vi "RecordingDisplay_171213.vi"(0 "TrackLength":dbl, 1 "Segments":bool, 2 "NormalMousebackgraound":picture, 4 "BackgroundSegments":picture, 6 "X":i32, 7 "Y":i32, 8 "i":i32, 9 "X in":i32[](array[numeric]), 10 "Angle":dbl, 11 "Y in":i32[](array[numeric])) -> (12 "X out":i32[](array[numeric]), 13 "Y out":i32[](array[numeric]), 19 "RecordingDisplay":picture)   [LabVIEW 2016]
uses:
  Globaltracker.vi
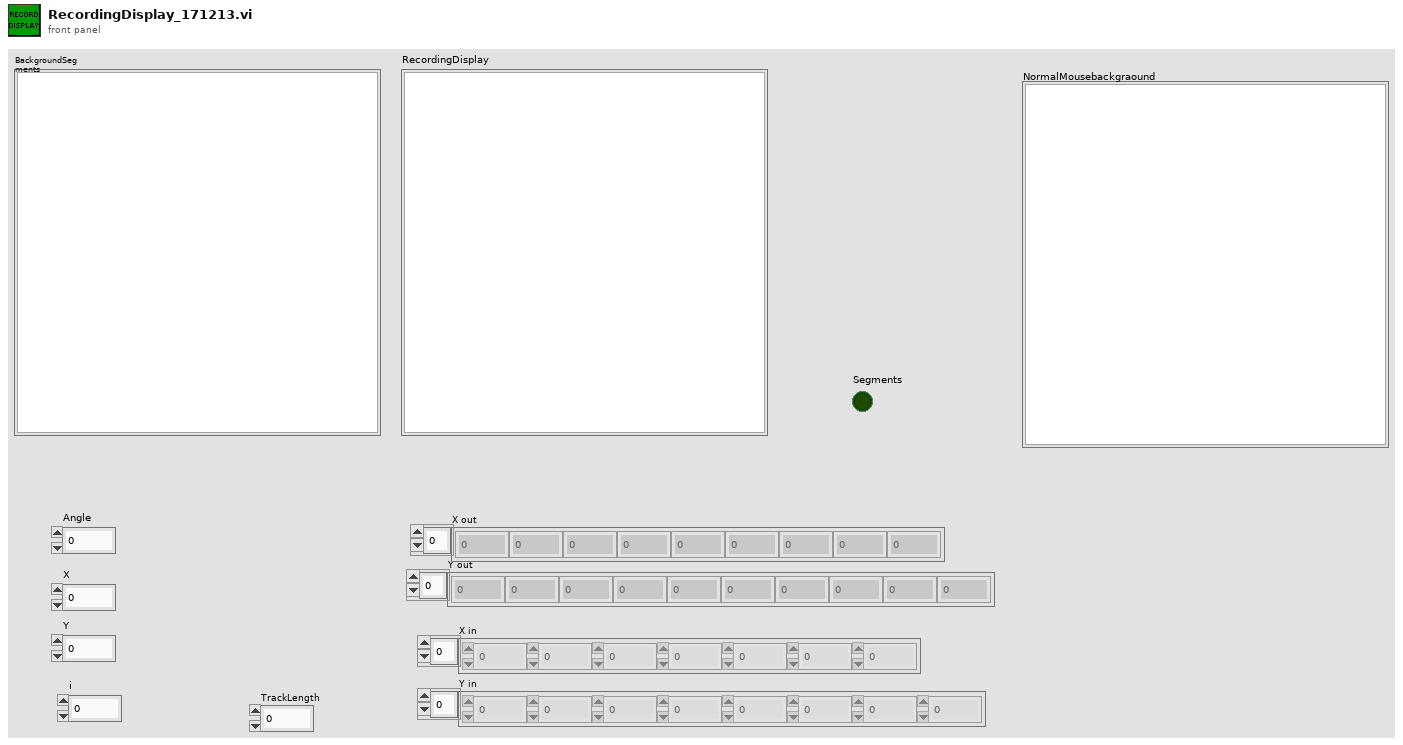
[diagram p1: front panel]
types:
  T1 = typedef "imagedata.ctl" = cluster{"image type":i32, "image depth":i32, "image":u8[], "mask":u8[], "colors":u32[], "Rectangle":cluster{"left":i16, "top":i16, "right":i16, "bottom":i16}}
  T2 = cluster{"left":i16, "top":i16, "right":i16, "bottom":i16}
  T3 = cluster{"image type":i32, "image depth":i32, "image":u8[], "mask":u8[], "colors":u32[], cluster{i32, i32, i32, i32}}
  T4 = cluster{"Width":u16, "Style":enum32{"Solid", "Dash", "Dot", "DashDot", "DashDotDot"}}
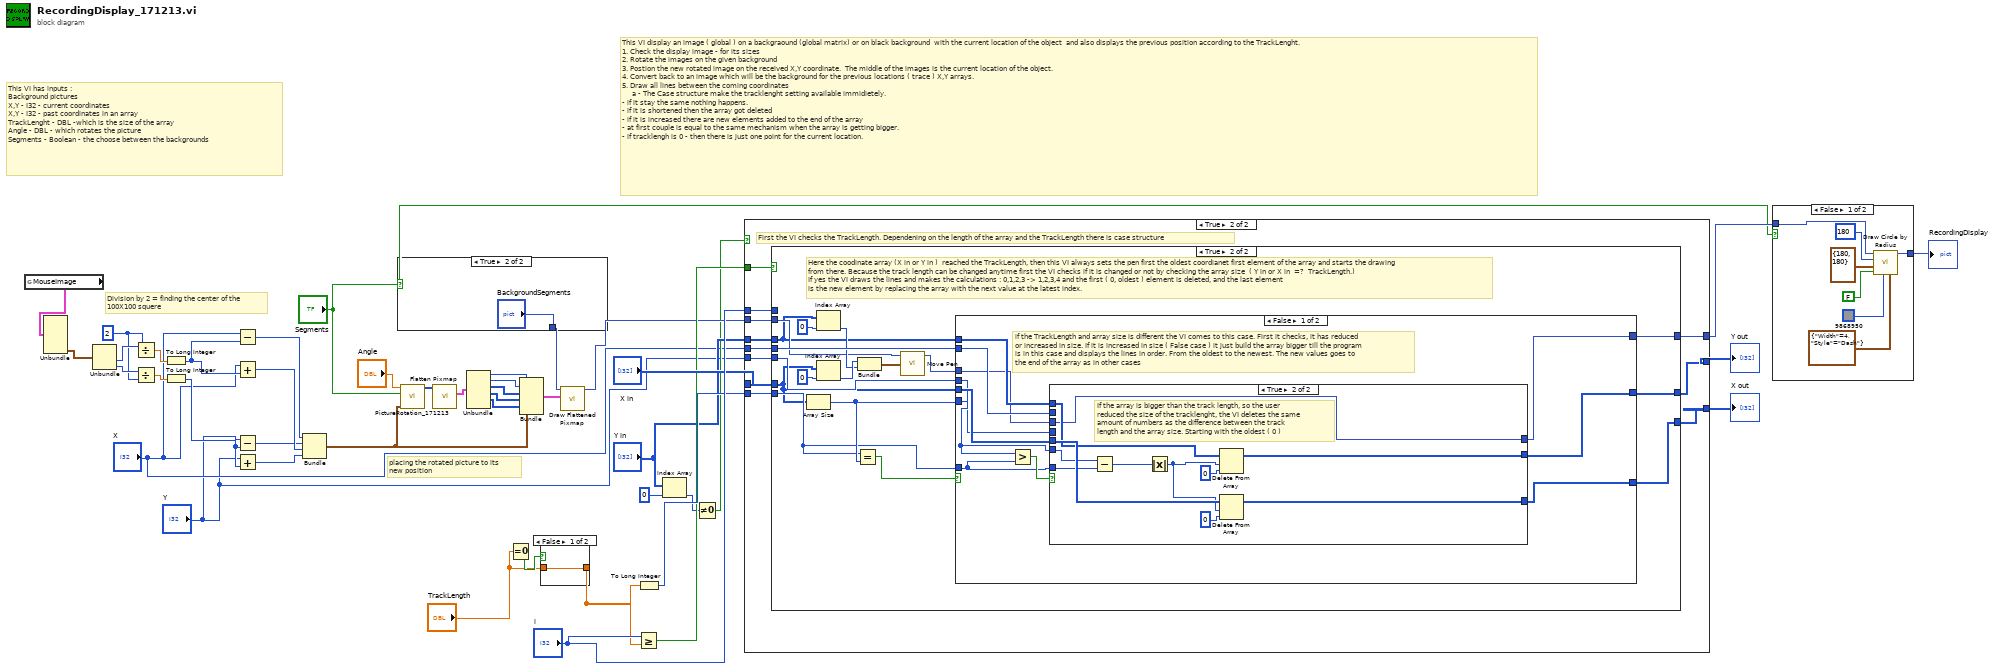
[diagram p0: block diagram]
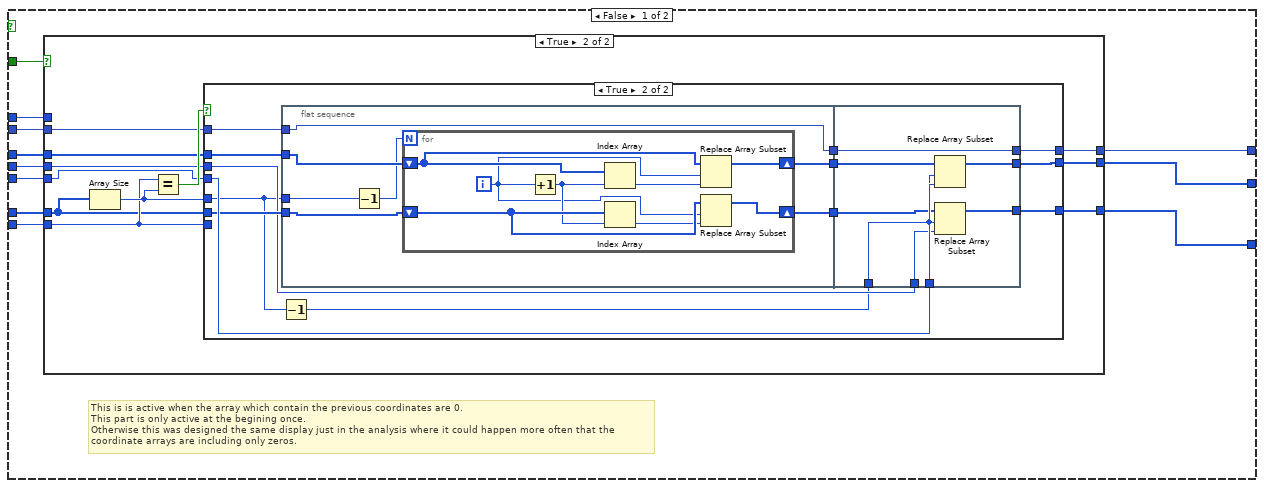
[diagram p2: hidden frame]
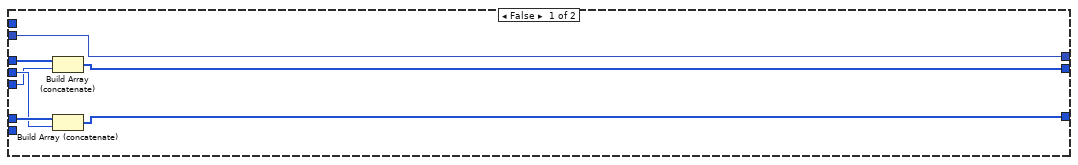
[diagram p3: hidden frame]
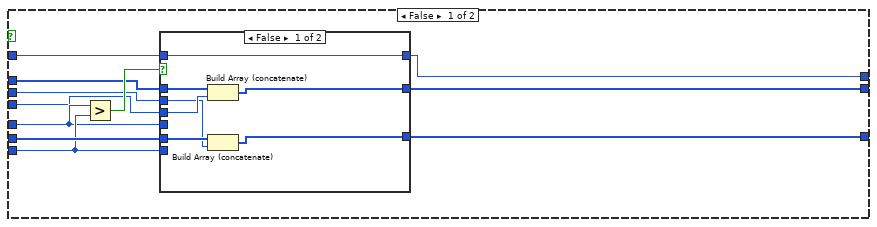
[diagram p4: hidden frame]
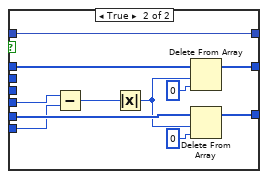
[diagram p5: hidden frame]
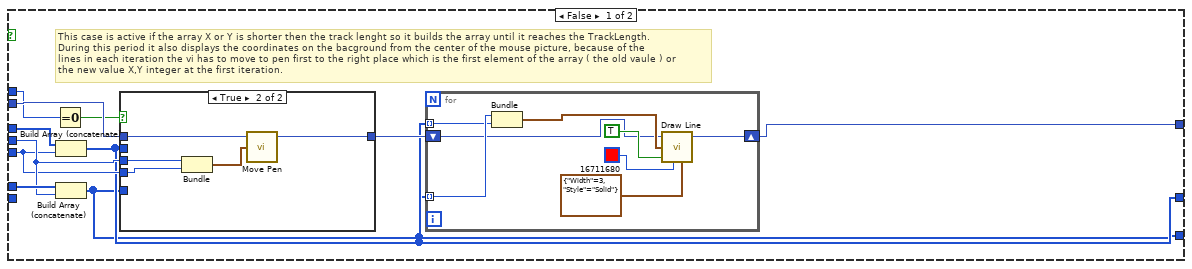
[diagram p6: hidden frame]
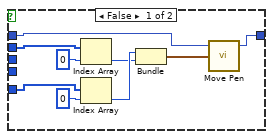
[diagram p7: hidden frame]
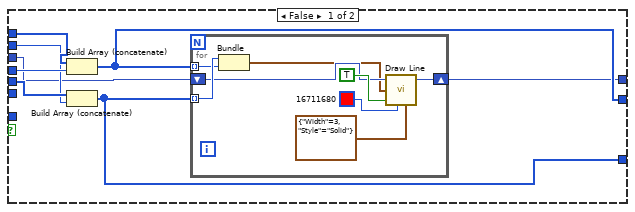
[diagram p8: hidden frame]
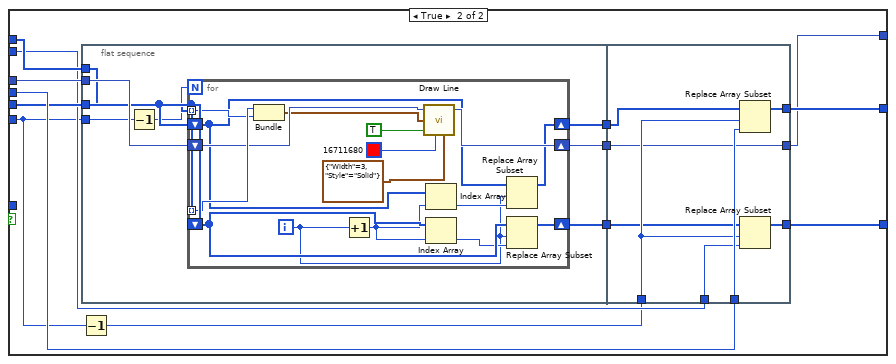
[diagram p9: hidden frame]
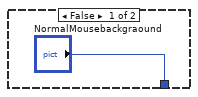
[diagram p10: hidden frame]
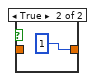
[diagram p11: hidden frame]
diagram:
  w17 = i16 2 ("y")
  # "placing the rotated picture to its \nnew position"
  # "Division by 2 = finding the center of the\n100X100 squere"
  # "This VI display an image ( global ) on a backgraound (global matrix) or on black background  with the current location of the object  and also displays the previous position according to the TrackLenght.\n1. Check the display image - for its sizes\n2. Rotate the images on the given background\n3. Postion the new rotated image on the received X,Y coordinate.  The middle of the images is the current location of the object.\n4. Convert back to an image which will be the background for the previous locations ( trace ) X,Y arrays. \n5. Draw all lines between the coming coordinates \n     a - The Case structure make the tracklenght setting available immidietely. \n- if it stay the same nothing happens.\n- if it is shortened then the array got deleted\n- if it is increased there are new elements added to the end of the array\n- at first couple is equal to the same mechanism when the array is getting bigger.\n- if tracklengh is 0 - then there is just one point for the current location."
  # "This VI has inputs : \nBackground pictures\nX,Y - I32 - current coordinates \nX,Y - I32 - past coordinates in an array \nTrackLenght - DBL -which is the size of the array\nAngle - DBL - which rotates the picture\nSegments - Boolean - the choose between the backgrounds"
  n1 = global read "Globaltracker.vi" "MouseImage"() -> (w21:T1)
  n2 = Unbundle(w21) -> ("Rectangle"=w20:T2)  [unwired: 5 out]
  n3 = Unbundle(w20) -> ("right"=w19:i16, "bottom"=w18:i16)  [unwired: 2 out]
  n4 = Divide(x=w19, y=w17) -> (x/y=w16:dbl)
  n5 = Divide(x=w18, y=w17) -> (x/y=w15:dbl)
  n6 = To Long Integer(number=w16) -> (32bit integer=w14:i32)
  n7 = To Long Integer(number=w15) -> (32bit integer=w13:i32)
  n8 = Subtract(x="X", y=w14) -> (x-y=w35:i32)
  n9 = Add(x="X", y=w14) -> (x+y=w34:i32)
  n10 = Subtract(x="Y", y=w13) -> (x-y=w32:i32)
  n11 = Add(x="Y", y=w13) -> (x+y=w33:i32)
  n12 = Bundle(w35, w32, w34, w33) -> (w24:cluster{i32, i32, i32, i32})  [unwired: 1 in]
  n13 = case shown="True" "Segments" {
    tunnel: ["NormalMousebackgraound" "BackgroundSegments"] -> w8
    frame False {
    }
    frame True {
    }
  }
  n14 = call "PictureRotation_171213.vi"("Cluster"=w24, "Segments"="Segments", "Angle"="Angle") -> ("Array"=w12:u32[][])  [unwired: 8 in]
  n15 = call <vilib>:"Flatten Pixmap.vi"("24-bit pixmap"=w12) -> ("image data"=w30:T1)  [unwired: 10 in]
  n16 = Unbundle(w30) -> ("image type"=w29:i32, "image depth"=w28:i32, "image"=w27:u8[], "mask"=w26:u8[], "colors"=w25:u32[])  [unwired: 1 out]
  n17 = Equal To 0?(x="TrackLength") -> (x = 0?=w42:bool)
  n18 = Bundle("image type"=w29, "image depth"=w28, "image"=w27, "mask"=w26, "colors"=w25, w24) -> (w23:T3)  [unwired: 1 in]
  n19 = case shown="False" w42 {
    tunnel: "TrackLength" -> [w46 _]
    tunnel: [w46 1] -> w7
    frame False {
    }
    frame True {
    }
  }
  n20 = call <vilib>:"Draw Flattened Pixmap.vi"("image data"=w23, "picture"=w8) -> ("new picture"=w22:picture)  [unwired: 7 in]
  n21 = Greater Or Equal?(x="i", y=w7) -> (x >= y?=w36:bool)
  n22 = To Long Integer(number=w7) -> (32bit integer=w40:i32)
  n23 = Index Array(array="Y in", index=0) -> (element=w5:i32)
  n24 = Not Equal To 0?(x=w5) -> (x != 0?=w3:bool)
  n25 = case shown="True" w3 {
    tunnel: "i" -> [w52 w152]
    tunnel: w40 -> [w53 w151]
    tunnel: "X in" -> [w57 w150]
    tunnel: [w48 w149] -> w38
    tunnel: [w49 w148] -> w37
    tunnel: w36 -> [w51 w147]
    tunnel: w22 -> [w58 w146]
    tunnel: [w50 w145] -> w11
    tunnel: "X" -> [w55 w144]
    tunnel: "Y" -> [w54 w143]
    tunnel: "Y in" -> [w56 w142]
    frame False {
      # "This is is active when the array which contain the previous coordinates are 0. \nThis part is only active at the begining once.\nOtherwise this was designed the same display just in the analysis where it could happen more often that the \ncoordinate arrays are including only zeros."
      n26 = case shown="True" w51 {
        tunnel: [w59 w75] -> w50
        tunnel: w52 -> [_ _]
        tunnel: w53 -> [_ w72]
        tunnel: w54 -> [w62 w71]
        tunnel: [w60 w69] -> w49
        tunnel: [w61 w76] -> w48
        tunnel: w56 -> [w65 w68]
        tunnel: w57 -> [w64 w67]
        tunnel: w55 -> [w63 w70]
        tunnel: w58 -> [w59 w66]
        frame False {
          n27 = Build Array (concatenate)(w65, w62) -> (w61:i32[])
          n28 = Build Array (concatenate)(w64, w63) -> (w60:i32[])
        }
        frame True {
          n29 = Array Size(array=w67) -> (size(s)=w73:i32)
          n30 = Equal?(x=w72, y=w73) -> (x = y?=w74:bool)
          n31 = case shown="True" w74 {
            tunnel: [w86 w118] -> w69
            tunnel: [w85 w117] -> w76
            tunnel: w71 -> [w77 w116]
            tunnel: w67 -> [w84 w115]
            tunnel: w68 -> [w83 w114]
            tunnel: w66 -> [w79 w113]
            tunnel: [w78 w109] -> w75
            tunnel: w73 -> [w81 w108]
            tunnel: w72 -> [w82 _]
            tunnel: w70 -> [w80 w112]
            frame False {
              n32 = Greater?(x=w81, y=w82) -> (0:w87:bool)
              n33 = case shown="False" w87 {
                tunnel: [w89 w105] -> w86
                tunnel: [w90 w104] -> w85
                tunnel: w84 -> [w94 w103]
                tunnel: w83 -> [w93 w102]
                tunnel: w81 -> [_ w101]
                tunnel: w82 -> [_ w97]
                tunnel: w77 -> [w92 _]
                tunnel: w80 -> [w91 _]
                tunnel: w79 -> [w88 w98]
                tunnel: [w88 w98] -> w78
                frame False {
                  n34 = Build Array (concatenate)(w93, w92) -> (w90:i32[])
                  n35 = Build Array (concatenate)(w94, w91) -> (w89:i32[])
                }
                frame True {
                  n36 = Subtract(x=w101, y=w97) -> (x-y=w100:i32)
                  n37 = Absolute Value(x=w100) -> (abs(x)=w99:i32)
                  n38 = Delete From Array(array=w102, length=w99, index=0) -> (array with subset deleted=w104:i32[])  [unwired: 1 out]
                  n39 = Delete From Array(array=w103, length=w99, index=0) -> (array with subset deleted=w105:i32[])  [unwired: 1 out]
                }
              }
            }
            frame True {
              n40 = Decrement(x=w108) -> (x-1=w111:i32)
              n41 = flat-sequence {
                tunnel: w115 -> [w125]
                tunnel: w114 -> [w124]
                tunnel: w113 -> [w119]
                tunnel: [w119] -> w110
                tunnel: w108 -> [w123]
                tunnel: [w121] -> w107
                tunnel: [w120] -> w106
                tunnel: [w141] -> w118
                tunnel: [w140] -> w117
                tunnel: w116 -> [w139]
                tunnel: w112 -> [w138]
                tunnel: w111 -> [w137]
                tunnel: w110 -> [w136]
                tunnel: [w136] -> w109
                tunnel: w107 -> [w135]
                tunnel: w106 -> [w134]
                frame #0 {
                  n42 = Decrement(x=w123) -> (x-1=w122:i32)
                  n43 = for {
                    N: w122 -> [_]
                    shift-right: [w127] -> w121
                    shift-left: w125 -> [w133]
                    shift-right: [w126] -> w120
                    shift-left: w124 -> [w132]
                    i -> [w128]
                    n44 = Increment(x=w128) -> (x+1=w131:i32)
                    n45 = Index Array(array=w132, index=w131) -> (element=w129:i32)
                    n46 = Index Array(array=w133, index=w131) -> (element=w130:i32)
                    n47 = Replace Array Subset(array=w132, new element=w129, index=w128) -> (w126:i32[])
                    n48 = Replace Array Subset(array=w133, new element=w130, index=w128) -> (w127:i32[])
                  }
                }
                frame #1 {
                  n49 = Replace Array Subset(array=w134, new element=w139, index=w137) -> (w140:i32[])
                  n50 = Replace Array Subset(array=w135, new element=w138, index=w137) -> (w141:i32[])
                }
              }
            }
          }
        }
      }
    }
    frame True {
      # "First the VI checks the TrackLength. Dependening on the length of the array and the TrackLength there is case structure"
      n51 = case shown="True" w147 {
        tunnel: [w161 w201] -> w145
        tunnel: w152 -> [w156 _]
        tunnel: w151 -> [_ w198]
        tunnel: w143 -> [w158 w197]
        tunnel: [w153 w195] -> w148
        tunnel: [w154 w202] -> w149
        tunnel: w142 -> [w163 w187]
        tunnel: w150 -> [w162 w186]
        tunnel: w144 -> [w160 w196]
        tunnel: w146 -> [w159 w189]
        frame False {
          # "This case is active if the array X or Y is shorter then the track lenght so it builds the array until it reaches the TrackLength.\nDuring this period it also displays the coordinates on the bacground from the center of the mouse picture, because of the \nlines in each iteration the vi has to move to pen first to the right place which is the first element of the array ( the old vaule ) or \nthe new value X,Y integer at the first iteration."
          n52 = Equal To 0?(x=w156) -> (x = 0?=w157:bool)
          n53 = Build Array (concatenate)(w163, w158) -> (w154:i32[])
          n54 = Build Array (concatenate)(w162, w160) -> (w153:i32[])
          n55 = case shown="True" w157 {
            tunnel: w160 -> [_ w177]
            tunnel: w159 -> [w170 w176]
            tunnel: w158 -> [_ w175]
            tunnel: [w171 w173] -> w155
            tunnel: w154 -> [w169 _]
            tunnel: w153 -> [w168 _]
            frame False {
              n56 = Index Array(array=w169, index=0) -> (element=w164:i32)
              n57 = Index Array(array=w168, index=0) -> (element=w165:i32)
              n58 = Bundle("X"=w165, "Y"=w164) -> (w172:cluster{"X":i32, "Y":i32})  [unwired: 1 in]
              n59 = call <vilib>:"Move Pen.vi"("new position"=w172, "picture"=w170) -> ("new picture"=w171:picture)  [unwired: 3 in]
            }
            frame True {
              n60 = Bundle("X"=w177, "Y"=w175) -> (w174:cluster{"X":i32, "Y":i32})  [unwired: 1 in]
              n61 = call <vilib>:"Move Pen.vi"("new position"=w174, "picture"=w176) -> ("new picture"=w173:picture)  [unwired: 3 in]
            }
          }
          n62 = for {
            tunnel: w153 -> [w185] mode=indexing
            tunnel: w154 -> [w184] mode=indexing
            shift-right: [w179] -> w161
            shift-left: w155 -> [w178]
            n63 = Bundle("X"=w185, "Y"=w184) -> (w180:cluster{"X":i32, "Y":i32})  [unwired: 1 in]
            n64 = call <vilib>:"Draw Line.vi"("picture"=w178, "end point"=w180, "absolute coordinates?(T)"=TRUE, "color(black)"=u32 16711680, "pen"=T4 {"Width"=3, "Style"=enum."Solid"}) -> ("new picture"=w179:picture)  [unwired: 4 in]
          }
        }
        frame True {
          # "Here the coodinate array (X in or Y in )  reached the TrackLength, then this VI always sets the pen first the oldest coordianet first element of the array and starts the drawing \nfrom there. Because the track length can be changed anytime first the VI checks if it is changed or not by checking the array size  ( Y in or X in  =?  TrackLength.)\nIf yes the VI draws the lines and makes the calculations : 0,1,2,3 -> 1,2,3,4 and the first ( 0, oldest ) element is deleted, and the last element\nis the new element by replacing the array with the next value at the latest index."
          n65 = Array Size(array=w186) -> (size(s)=w199:i32)
          n66 = Index Array(array=w187, index=0) -> (element=w192:i32)
          n67 = Index Array(array=w186, index=0) -> (element=w193:i32)
          n68 = Equal?(x=w198, y=w199) -> (x = y?=w200:bool)
          n69 = Bundle(w193, w192) -> (w194:cluster{i32, i32})  [unwired: 1 in]
          n70 = call <vilib>:"Move Pen.vi"("new position"=w194, "picture"=w189) -> ("new picture"=w188:picture)  [unwired: 3 in]
          n71 = case shown="False" w200 {
            tunnel: [w212 w253] -> w195
            tunnel: [w211 w252] -> w202
            tunnel: w197 -> [w203 w251]
            tunnel: w186 -> [w210 w250]
            tunnel: w187 -> [w209 w249]
            tunnel: w188 -> [w205 w248]
            tunnel: [w204 w244] -> w201
            tunnel: w199 -> [w207 w243]
            tunnel: w198 -> [w208 _]
            tunnel: w196 -> [w206 w247]
            frame False {
              # "if the TrackLength and array size is different the VI comes to this case. First it checks, it has reduced\nor increased in size. If it is increased in size ( False case ) it just build the array bigger till the program\nis in this case and displays the lines in order. From the oldest to the newest. The new values goes to\nthe end of the array as in other cases"
              n72 = Greater?(x=w207, y=w208) -> (0:w213:bool)
              n73 = case shown="True" w213 {
                tunnel: [w216 w240] -> w212
                tunnel: [w217 w239] -> w211
                tunnel: w210 -> [w221 w238]
                tunnel: w209 -> [w220 w237]
                tunnel: w207 -> [_ w236]
                tunnel: w208 -> [_ w232]
                tunnel: w203 -> [w219 _]
                tunnel: w206 -> [w218 _]
                tunnel: w205 -> [w215 w233]
                tunnel: [w214 w233] -> w204
                frame False {
                  n74 = Build Array (concatenate)(w220, w219) -> (w217:i32[])
                  n75 = Build Array (concatenate)(w221, w218) -> (w216:i32[])
                  n76 = for {
                    tunnel: w216 -> [w229] mode=indexing
                    tunnel: w217 -> [w228] mode=indexing
                    shift-right: [w222] -> w214
                    shift-left: w215 -> [w224]
                    n77 = Bundle("X"=w229, "Y"=w228) -> (w223:cluster{"X":i32, "Y":i32})  [unwired: 1 in]
                    n78 = call <vilib>:"Draw Line.vi"("picture"=w224, "end point"=w223, "absolute coordinates?(T)"=TRUE, "color(black)"=u32 16711680, "pen"=T4 {"Width"=3, "Style"=enum."Solid"}) -> ("new picture"=w222:picture)  [unwired: 4 in]
                  }
                }
                frame True {
                  # "If the array is bigger than the track length, so the user\nreduced the size of the tracklenght, the VI deletes the same\namount of numbers as the difference between the track\nlength and the array size. Starting with the oldest ( 0 )"
                  n79 = Subtract(x=w236, y=w232) -> (x-y=w235:i32)
                  n80 = Absolute Value(x=w235) -> (abs(x)=w234:i32)
                  n81 = Delete From Array(array=w237, length=w234, index=0) -> (array with subset deleted=w239:i32[])  [unwired: 1 out]
                  n82 = Delete From Array(array=w238, length=w234, index=0) -> (array with subset deleted=w240:i32[])  [unwired: 1 out]
                }
              }
            }
            frame True {
              n83 = Decrement(x=w243) -> (x-1=w246:i32)
              n84 = flat-sequence {
                tunnel: w250 -> [w259]
                tunnel: w249 -> [w258]
                tunnel: w248 -> [w261]
                tunnel: [w260] -> w245
                tunnel: w243 -> [w257]
                tunnel: [w255] -> w242
                tunnel: [w254] -> w241
                tunnel: [w285] -> w253
                tunnel: [w284] -> w252
                tunnel: w251 -> [w283]
                tunnel: w247 -> [w282]
                tunnel: w246 -> [w281]
                tunnel: w245 -> [w280]
                tunnel: [w280] -> w244
                tunnel: w242 -> [w279]
                tunnel: w241 -> [w278]
                frame #0 {
                  n85 = Decrement(x=w257) -> (x-1=w256:i32)
                  n86 = for {
                    N: w256 -> [_]
                    tunnel: w259 -> [w277] mode=indexing
                    tunnel: w258 -> [w276] mode=indexing
                    shift-right: [w270] -> w260
                    shift-left: w261 -> [w272]
                    shift-right: [w263] -> w255
                    shift-left: w259 -> [w269]
                    shift-right: [w262] -> w254
                    shift-left: w258 -> [w268]
                    i -> [w264]
                    n87 = Bundle(w277, w276) -> (w271:cluster{i32, i32})  [unwired: 1 in]
                    n88 = Increment(x=w264) -> (x+1=w267:i32)
                    n89 = call <vilib>:"Draw Line.vi"("picture"=w272, "end point"=w271, "absolute coordinates?(T)"=TRUE, "color(black)"=u32 16711680, "pen"=T4 {"Width"=3, "Style"=enum."Solid"}) -> ("new picture"=w270:picture)  [unwired: 4 in]
                    n90 = Index Array(array=w268, index=w267) -> (element=w265:i32)
                    n91 = Index Array(array=w269, index=w267) -> (element=w266:i32)
                    n92 = Replace Array Subset(array=w268, new element=w265, index=w264) -> (w262:i32[])
                    n93 = Replace Array Subset(array=w269, new element=w266, index=w264) -> (w263:i32[])
                  }
                }
                frame #1 {
                  n94 = Replace Array Subset(array=w278, new element=w283, index=w281) -> (w284:i32[])
                  n95 = Replace Array Subset(array=w279, new element=w282, index=w281) -> (w285:i32[])
                }
              }
            }
          }
        }
      }
    }
  }
  "Y out" <- w38
  "X out" <- w37
  n96 = case shown="False" "Segments" {
    tunnel: w11 -> [w290 w293]
    tunnel: [w289 w293] -> w10
    frame False {
      n97 = call <vilib>:"Draw Circle by Radius.vi"("pen"=T4 {"Width"=4, "Style"=enum."Dash"}, "color(black)"=u32 9868950, "fill?(F)"=FALSE, "pixel center"=cluster{"horizontal":i16, "vertical":i16} {"horizontal"=180, "vertical"=180}, "radius"=i16 180, "picture"=w290) -> ("new picture"=w289:picture)  [unwired: 5 in]
    }
    frame True {
    }
  }
  "RecordingDisplay" <- w10
